vi "Variant to Header Info.vi"(4 "Variant":refnum<class "variant.lvclass">) -> (0 "Type Descriptor Header":T1 {"type" format="%.0x"}, 1 "TypeDescriptor":refnum<class "TD.lvclass">, 5 "DataString":refnum<class "DataString.lvclass">)   [LabVIEW 2020, in "variant.lvlib" / "variant.lvclass"]
doc: "Returns flattened string and type descriptor of variant data, plus selected type info."
uses:
  Type Descriptor Header.ctl
  Type Descriptor Enumeration.ctl
  variant.lvclass
  variant.lvclass/variant.ctl
  Type Descriptor/TD.lvclass
  openg_variant.lvlib
  DataString/DataString.lvclass
panel:
  # "[OpenG VI Tags] ***Do Not Remove***"
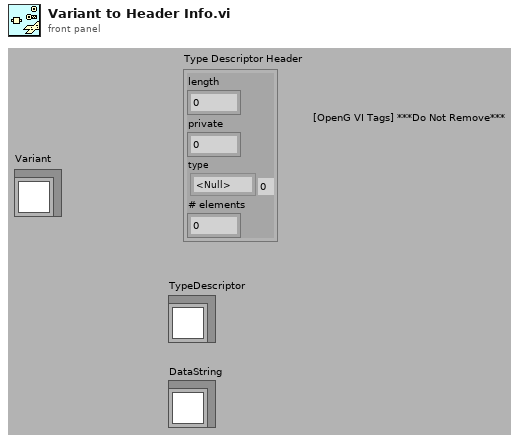
[diagram p1: front panel]
types:
  T1 = typedef "openg_variant.lvlib/Type Descriptor Header.ctl" = cluster{"length":u16, "private":u8, "type":T2, "# elements":u16}
  T2 = typedef "openg_variant.lvlib/Type Descriptor Enumeration.ctl" = enum8{"<Null>", "I8", "I16", "I32", "I64", "U8", "U16", "U32", "U64", "SGL", "DBL", "EXT", "CSG", "CDB", "CXT", "0x0F", "0x10", "0x11", "0x12", "0x13", "0x14", "Enum U8", "Enum U16", "Enum U32", "Enum U64", "SGL PQ", "DBL PQ", "EXT PQ", "CSG PQ", "CDB PQ", "CXT PQ", "0x1F", "0x20", "Boolean", "0x22", "0x23", "0x24", "0x25", "0x26", "0x27", "0x28", "0x29", "0x2A", "0x2B", "0x2C", "0x2D", "0x2E", "0x2F", "String", "0x31", "Path", "Pict", "0x34", "0x35", "0x36", "DAQ", "0x38", "0x39", "0x3A", "0x3B", "0x3C", "0x3D", "0x3E", "0x3F", "Array", "0x41", "0x42", "0x43", "0x44", "0x45", "0x46", "0x47", "0x48", "0x49", "0x4A", "0x4B", "0x4C", "0x4D", "0x4E", "0x4F", "Cluster", "0x51", "0x52", "Variant", "Waveform", "0x55", "0x56", "0x57", "0x58", "0x59", "0x5A", "0x5B", "0x5C", "0x5D", "0x5E", "Fixed Point", "0x60", "0x61", "0x62", "0x63", "0x64", "0x65", "0x66", "0x67", "0x68", "0x69", "0x6A", "0x6B", "0x6C", "0x6D", "0x6E", "0x6F", "Refnum", "0x71", "0x72", "Set Collection", "Map Collection"}
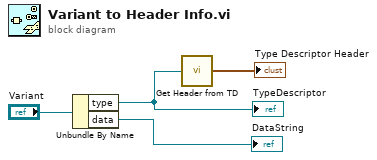
[diagram p0: block diagram]
diagram:
  n1 = Unbundle By Name("Variant") -> ("type"=w2:refnum<class "TD.lvclass">, "data"=→"DataString":refnum<class "DataString.lvclass">)
  "TypeDescriptor" <- w2
  n2 = call "Get Header from TD.vi"("TypeDescriptor"=w2) -> ("Type Descriptor Header"=→"Type Descriptor Header":T1)
